vi "Test-RawAssemblyCalls.vi"() -> ()   [LabVIEW 2015]
uses:
  C:/Users/Public/Documents/Projects/lv-winscp/Bin WinSCP/WinSCPnet.dll
  Bin WinSCP/WinSCPnet.dll
panel:
  out "ExitCode":i32
  out "ErrorOutput":string
  out "IsSuccess 2":bool
  out "Output":string
  out "Array 3":cluster{"Message":string, "Source":string}[](array[cluster])
  out "Array 2":T1(array[cluster])
  out "IsSuccess":bool
  out "Count":i32
  out "Array":T2(array[cluster])
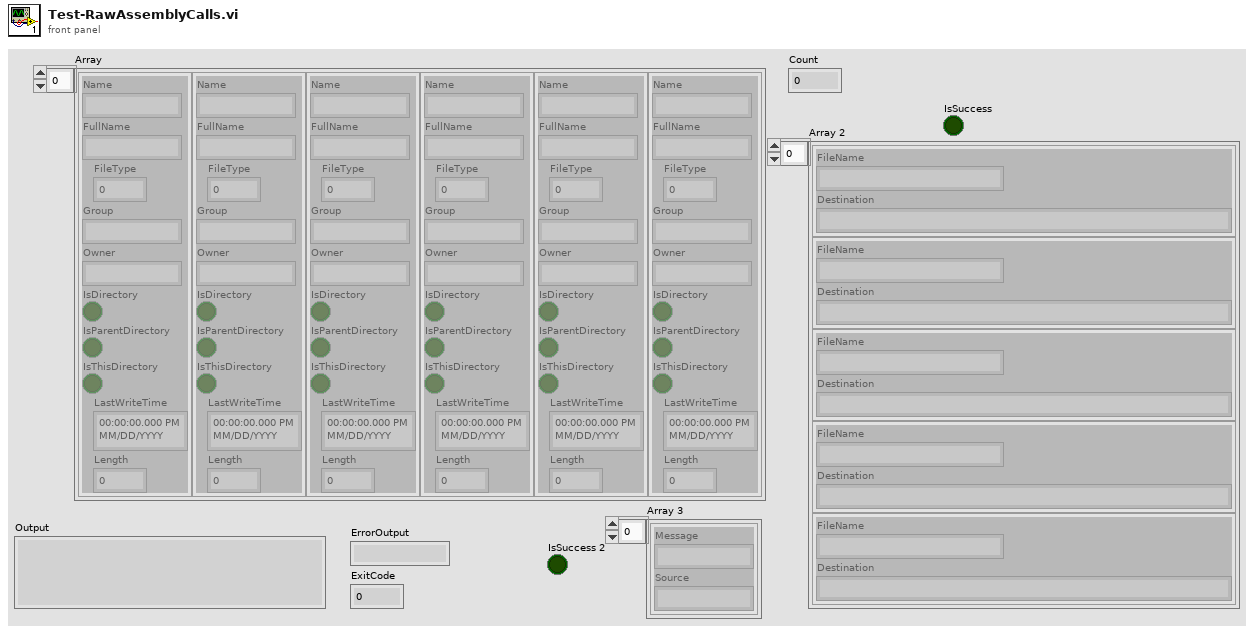
[diagram p1: front panel]
types:
  T1 = cluster{"FileName":string, "Destination":string}[]
  T2 = cluster{"Name":string, "FullName":string, "FileType":u16, "Group":string, "Owner":string, "IsDirectory":bool, "IsParentDirectory":bool, "IsThisDirectory":bool, "LastWriteTime":timestamp, "Length":i64}[]
  T3 = cluster{"Name":string, "FullName":string, "FileType":u16, "Group":string, "Owner":string, "IsDirectory":bool, "IsParentDirectory":bool, "IsThisDirectory":bool, "LastWriteTime":timestamp, "Length":i64}
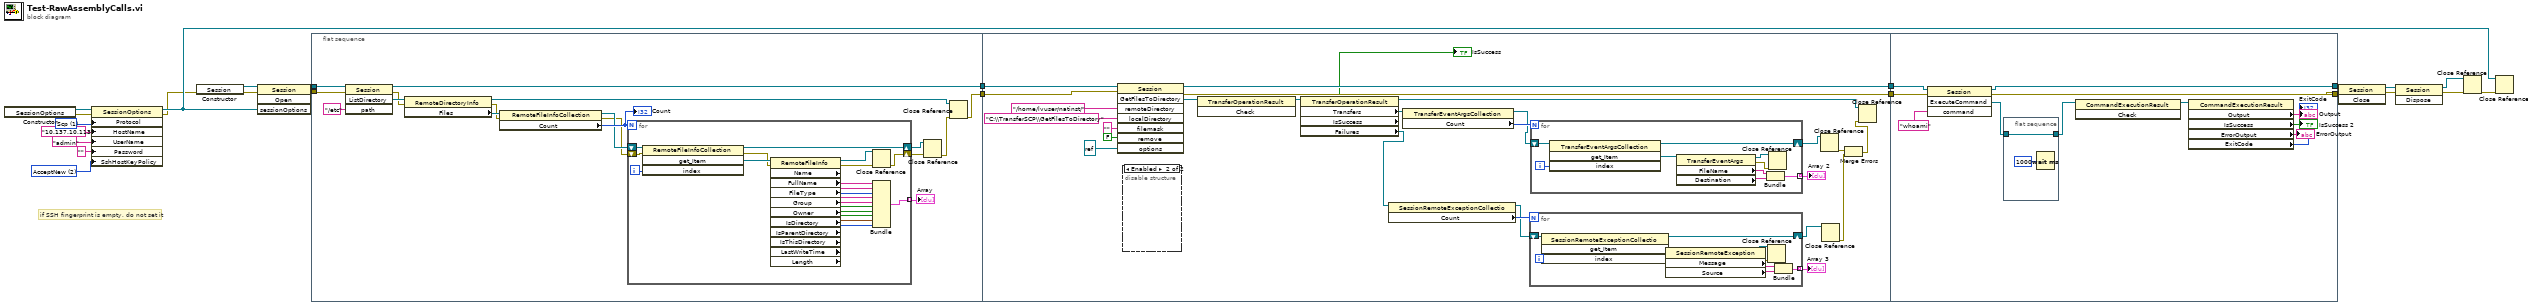
[diagram p0: block diagram]
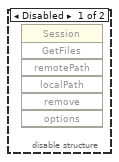
[diagram p2: hidden frame]
diagram:
  w21 = 2 items=["Check", "GiveUpSecurityAndAcceptAny", "AcceptNew"] ("SshHostKeyPolicy")
  w22 = 1 items=["Sftp", "Scp", "Ftp", "Webdav", "S3"] ("Protocol")
  # "if SSH fingerprint is empty, do not set it"
  n1 = constructor class="SessionOptions"() -> (reference out=w24:refnum<k24>, error out=w23:errorcluster)  [unwired: 3 in, 1 out]
  n2 = property class="SessionOptions"(reference=w24, error in=w23, "Protocol"=w22, "HostName"="10.137.10.113", "UserName"="admin", "Password"="", "SshHostKeyPolicy"=w21) -> (reference out=w9:refnum<k24>, error out=w8:errorcluster)
  n3 = constructor class="Session"(error in=w8) -> (reference out=w17:refnum<k24>, error out=w7:errorcluster)  [unwired: 2 in, 1 out]
  n4 = invoke class="Session" method="Open"(reference=w17, error in=w7, "sessionOptions"=w9) -> (reference out=w16:refnum<k24>, error out=w5:errorcluster)  [unwired: 1 in, 2 out]
  n5 = flat-sequence {
    tunnel: w16 -> [w41]
    tunnel: w5 -> [w40]
    tunnel: [w39] -> w4
    tunnel: [w25] -> w3
    tunnel: w4 -> [w87]
    tunnel: w3 -> [w85]
    tunnel: [w86] -> w2
    tunnel: [w84] -> w1
    tunnel: [w114] -> w6
    tunnel: [w116] -> w15
    tunnel: w2 -> [w117]
    tunnel: w1 -> [w115]
    frame #0 {
      n6 = invoke class="Session" method="ListDirectory"(reference=w41, error in=w40, "path"="/etc") -> (reference out=w39:refnum<k24>, error out=w27:errorcluster, "ListDirectory"=w37:refnum<k24>)  [unwired: 1 in, 1 out]
      n7 = property class="RemoteDirectoryInfo"(reference=w37, error in=w27) -> (reference out=w28:refnum<k24>, error out=w26:errorcluster, "Files"=w36:refnum<k24>)
      n8 = property class="RemoteFileInfoCollection"(reference=w36, error in=w26) -> (reference out=w34:refnum<k24>, error out=w33:errorcluster, "Count"=w35:i32)
      "Count" <- w35
      n9 = for {
        N: w35 -> [_]
        shift-right: [w61] -> w30
        shift-left: w34 -> [w60]
        tunnel: [w48] -> w32 mode=indexing
        shift-right: [w43] -> w31
        shift-left: w33 -> [w45]
        i -> [w42]
        n10 = invoke class="RemoteFileInfoCollection" method="get_Item"(reference=w60, error in=w45, "index"=w42) -> (reference out=w61:refnum<k24>, error out=w44:errorcluster, "get_Item"=w59:refnum<k24>)  [unwired: 1 in, 1 out]
        n11 = property class="RemoteFileInfo"(reference=w59, error in=w44) -> (reference out=w47:refnum<k24>, error out=w46:errorcluster, "Name"=w58:string, "FullName"=w57:string, "FileType"=w56:u16, "Group"=w55:string, "Owner"=w54:string, "IsDirectory"=w53:bool, "IsParentDirectory"=w52:bool, "IsThisDirectory"=w51:bool, "LastWriteTime"=w50:timestamp, "Length"=w49:i64)
        n12 = Close Reference(reference=w47, error in (no error)=w46) -> (error out=w43:errorcluster)
        n13 = Bundle("Name"=w58, "FullName"=w57, "FileType"=w56, "Group"=w55, "Owner"=w54, "IsDirectory"=w53, "IsParentDirectory"=w52, "IsThisDirectory"=w51, "LastWriteTime"=w50, "Length"=w49) -> (w48:T3)  [unwired: 1 in]
      }
      "Array" <- w32
      n14 = Close Reference(reference=w30, error in (no error)=w31) -> (error out=w29:errorcluster)
      n15 = Close Reference(reference=w28, error in (no error)=w29) -> (error out=w25:errorcluster)
    }
    frame #1 {
      n16 = invoke class="Session" method="GetFilesToDirectory"(reference=w87, error in=w85, "remoteDirectory"="/home/lvuser/natinst/" ("remotePath"), "localDirectory"="C:\\TransferSCP\\GetFilesToDirectory" ("localPath"), "filemask"="", "remove"=FALSE, "options"=refnum<k24> refnum) -> (reference out=w86:refnum<k24>, error out=w84:errorcluster, "GetFilesToDirectory"=w78:refnum<k24>)  [unwired: 1 in, 5 out]
      n17 = disable-structure shown="Enabled" {
        frame Disabled {
          n18 = invoke class="Session" method="GetFiles"() -> ()  [unwired: 7 in, 7 out]
        }
        frame Enabled {
        }
      }
      n19 = invoke class="TransferOperationResult" method="Check"(reference=w78) -> (reference out=w77:refnum<k24>)  [unwired: 2 in, 2 out]
      n20 = property class="TransferOperationResult"(reference=w77) -> (reference out=w70:refnum<k24>, "Transfers"=w76:refnum<k24>, "IsSuccess"=→"IsSuccess":bool, "Failures"=w69:refnum<k24>)  [unwired: 1 in, 1 out]
      n21 = property class="SessionRemoteExceptionCollectio"(reference=w69) -> (reference out=w67:refnum<k24>, "Count"=w68:i32)  [unwired: 1 in, 1 out]
      n22 = property class="TransferEventArgsCollection"(reference=w76) -> (reference out=w73:refnum<k24>, "Count"=w75:i32)  [unwired: 1 in, 1 out]
      n23 = for {
        N: w68 -> [_]
        shift-right: [w91] -> w65
        shift-left: w67 -> [w96]
        tunnel: [w90] -> w66 mode=indexing
        i -> [w95]
        n24 = invoke class="SessionRemoteExceptionCollectio" method="get_Item"(reference=w96, "index"=w95) -> (reference out=w91:refnum<k24>, "get_Item"=w94:refnum<k24>)  [unwired: 2 in, 2 out]
        n25 = property class="SessionRemoteException"(reference=w94) -> (reference out=w88:refnum<k24>, error out=w89:errorcluster, "Message"=w93:string, "Source"=w92:string)  [unwired: 1 in]
        n26 = Close Reference(reference=w88, error in (no error)=w89) -> ()  [unwired: 1 out]
        n27 = Bundle("Message"=w93, "Source"=w92) -> (w90:cluster{"Message":string, "Source":string})  [unwired: 1 in]
      }
      "Array 3" <- w66
      n28 = for {
        N: w75 -> [_]
        shift-right: [w100] -> w71
        shift-left: w73 -> [w105]
        tunnel: [w99] -> w72 mode=indexing
        i -> [w104]
        n29 = invoke class="TransferEventArgsCollection" method="get_Item"(reference=w105, "index"=w104) -> (reference out=w100:refnum<k24>, "get_Item"=w103:refnum<k24>)  [unwired: 2 in, 2 out]
        n30 = property class="TransferEventArgs"(reference=w103) -> (reference out=w97:refnum<k24>, error out=w98:errorcluster, "FileName"=w102:string, "Destination"=w101:string)  [unwired: 1 in]
        n31 = Bundle("FileName"=w102, "Destination"=w101) -> (w99:cluster{"FileName":string, "Destination":string})  [unwired: 1 in]
        n32 = Close Reference(reference=w97, error in (no error)=w98) -> ()  [unwired: 1 out]
      }
      "Array 2" <- w72
      n33 = Close Reference(reference=w71) -> (error out=w64:errorcluster)  [unwired: 1 in]
      n34 = Close Reference(reference=w65) -> (error out=w63:errorcluster)  [unwired: 1 in]
      n35 = Merge Errors(w64, w63) -> (w62:errorcluster)
      n36 = Close Reference(reference=w70, error in (no error)=w62) -> ()  [unwired: 1 out]
    }
    frame #2 {
      n37 = invoke class="Session" method="ExecuteCommand"(reference=w117, error in=w115, "command"="whoami") -> (reference out=w116:refnum<k24>, error out=w114:errorcluster, "ExecuteCommand"=w108:refnum<k24>)  [unwired: 1 in, 1 out]
      n38 = flat-sequence {
        tunnel: [w118] -> w107
        tunnel: w108 -> [w118]
        frame #0 {
          n39 = Wait (ms)(milliseconds to wait=u32 1000) -> ()  [unwired: 1 out]
        }
      }
      n40 = invoke class="CommandExecutionResult" method="Check"(reference=w107) -> (reference out=w109:refnum<k24>)  [unwired: 2 in, 2 out]
      n41 = property class="CommandExecutionResult"(reference=w109) -> ("Output"=→"Output":string, "IsSuccess"=→"IsSuccess 2":bool, "ErrorOutput"=→"ErrorOutput":string, "ExitCode"=→"ExitCode":i32)  [unwired: 1 in, 2 out]
    }
  }
  n42 = invoke class="Session" method="Close"(reference=w15, error in=w6) -> (reference out=w14:refnum<k24>, error out=w13:errorcluster)  [unwired: 1 in, 1 out]
  n43 = invoke class="Session" method="Dispose"(reference=w14, error in=w13) -> (reference out=w11:refnum<k24>, error out=w12:errorcluster)  [unwired: 1 in, 1 out]
  n44 = Close Reference(reference=w11, error in (no error)=w12) -> (error out=w10:errorcluster)
  n45 = Close Reference(reference=w9, error in (no error)=w10) -> ()  [unwired: 1 out]
